vi "Enable_Baxter.vi"(0 "error in":errorcluster, 2 "Enable?":bool=TRUE, 3 "node":string) -> (1 "error out":errorcluster)   [LabVIEW 2012]
doc: "This will enable all the motors on Baxter"
uses:
  <userlib>/ROSforLV/ROS/Code/Console/Servers/ServerSubs/TopicDef.ctl
  <userlib>/ROSforLV/ROS/Code/SubVIs/_ROSDirection.ctl
  <userlib>/ROSforLV/ROS/MessageBuilding/std_msgs/subs/boolScalar.vi
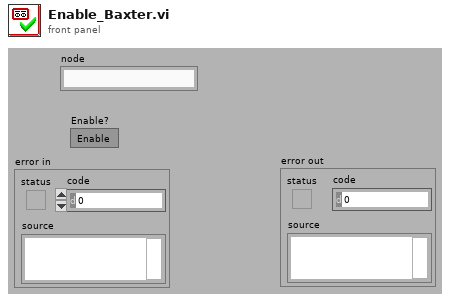
[diagram p1: front panel]
types:
  T1 = typedef "TopicDef.ctl" = cluster{"Topic":string, "Type":string, "Action":T2, "Update (ms)":u16, "queue size":u16}
  T2 = typedef "_ROSDirection.ctl" = enum16{"Node", "Publisher", "Subscriber", "Service Client"}
  T3 = typedef "_ROSControl.ctl" = cluster{"topic port":u16, "Node":string, "topic":string, "type":string, "node port":u16, "error ":errorcluster, "Direction":T2, "Update (ms)":u16, "queue size":u16}
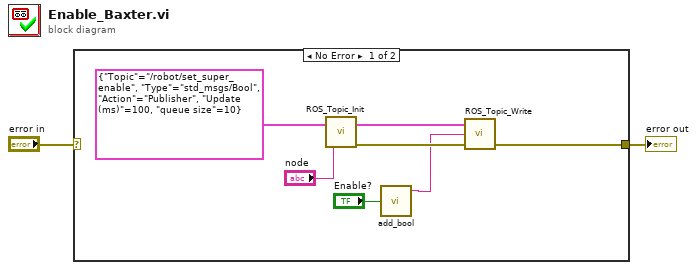
[diagram p0: block diagram]
diagram:
  n1 = case shown="No Error" "error in" {
    selector: "error in" -> [_ w10]
    tunnel: [w3 w10] -> w2
    frame No Error {
      n2 = call <userlib>:"ROS_Topic_Init.vi"("node"="node", "Definitions"=T1 {"Topic"="/robot/set_super_enable", "Type"="std_msgs/Bool", "Action"=enum."Publisher", "Update (ms)"=100, "queue size"=10}) -> ("error out"=w5:errorcluster, "ROS out"=w9:T3)
      n3 = call-poly <userlib>:"add_bool.vi"("Boolean"="Enable?") -> ("msg out"=w4:string)  [unwired: 4 in]
      n4 = call <userlib>:"ROS_Topic_Write.vi"("error in (no error)"=w5, "Msg in"=w4, "ROS in"=w9) -> ("error out"=w3:errorcluster)  [unwired: 1 in, 1 out]
    }
    frame Error {
    }
  }
  "error out" <- w2
